vi "Init Discovery Service.vi"(8 "error in (no error)":errorcluster, 11 "Vecto in":refnum<class "Vecto.lvclass">) -> (0 "error out":errorcluster, 3 "Vecto out":refnum<class "Vecto.lvclass">)   [LabVIEW 2020, in "Vecto.lvlib" / "Vecto.lvclass"]
uses:
  Vecto.lvclass
  Event Level.ctl
  Vecto.lvclass/Vecto.ctl
  EventLoggingService/EventLoggingService.lvclass/EventLoggingService.ctl
  <vilib>/Utility/error.llb/Error Cluster From Error Code.vi
  EventLogHandler/EventLogHandler.lvclass
  DiscoveryService/DiscoveryService.lvclass
  Vecto.lvlib
  Node Config/Node Config.lvclass
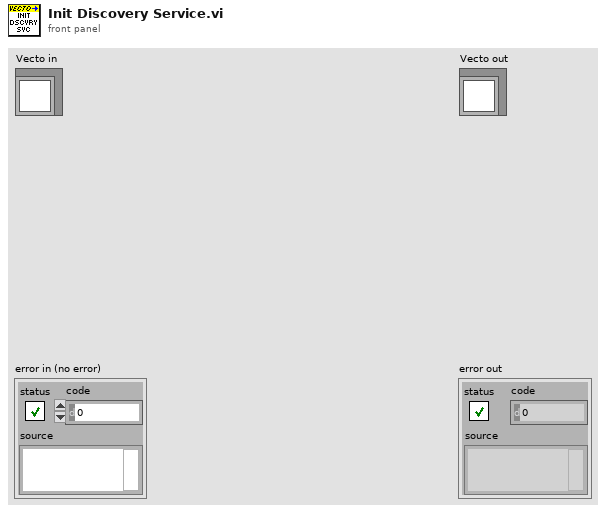
[diagram p1: front panel]
types:
  T1 = typedef "VectoConfig.lvlib/Comms Features.ctl" = cluster{"HTTP Server":bool, "TCP Messaging":bool, "Remote Data":bool, "Discovery":bool}
  T2 = typedef "Vecto.lvlib/Event Level.ctl" = enum16{"Debug", "Info", "Warning", "Error"}
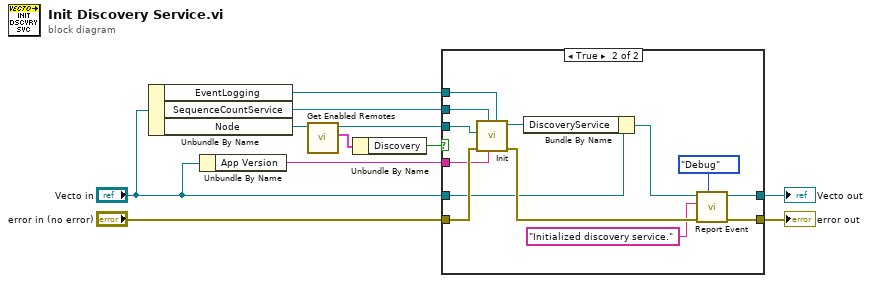
[diagram p0: block diagram]
diagram:
  n1 = Unbundle By Name("Vecto in") -> ("EventLogging"=w7:refnum<class "EventLoggingService.lvclass">, "SequenceCountService"=w10:refnum<class "SequenceCountService.lvclass">, "Node"=w4:refnum<class "Node Config.lvclass">)
  n2 = Unbundle By Name("Vecto in") -> ("App Version"=w8:string)
  n3 = call "Get Enabled Remotes.vi"("Node Config in"=w4) -> ("Comms Features"=w2:T1, "Node Config out"=w3:refnum<class "Node Config.lvclass">)  [unwired: 8 in, 1 out]
  n4 = Unbundle By Name(w2) -> ("Discovery"=w1:bool)
  n5 = case shown="True" w1 {
    tunnel: "error in (no error)" -> [w12 w25]
    tunnel: w10 -> [_ w23]
    tunnel: "Vecto in" -> [w13 w22]
    tunnel: w8 -> [_ w21]
    tunnel: w7 -> [_ w20]
    tunnel: [w12 w19] -> w6
    tunnel: [w13 w17] -> w5
    tunnel: w3 -> [_ w14]
    frame False {
    }
    frame True {
      n6 = call "Init.vi"("EventLogger"=w20, "App Version"=w21, "SequenceCountService"=w23, "error in (no error)"=w25, "Node"=w14) -> ("error out"=w26:errorcluster, "DiscoveryService out"=w24:refnum<class "DiscoveryService.lvclass">)  [unwired: 5 in]
      n7 = Bundle By Name(cluster=w22, "DiscoveryService"=w24) -> (w18:refnum<class "Vecto.lvclass">)
      n8 = call "Report Event.vi"("Event Level (Info)"=Event_Level."Debug", "error in (no error)"=w26, "Message"="Initialized discovery service.", "Vecto in"=w18) -> ("error out"=w19:errorcluster, "Vecto out"=w17:refnum<class "Vecto.lvclass">)  [unwired: 6 in]
    }
  }
  "error out" <- w6
  "Vecto out" <- w5
